vi "First_Num_from_String.vi"(1 "string":string) -> (0 "number":dbl)   [LabVIEW 2012]
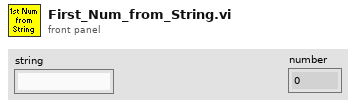
[diagram p1: front panel]
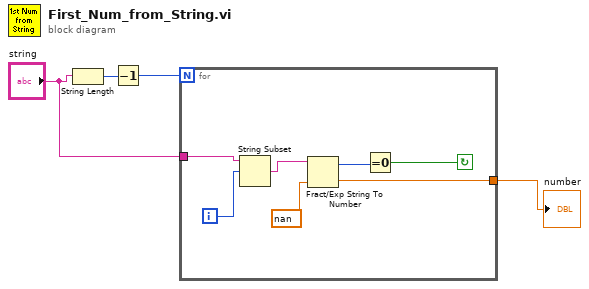
[diagram p0: block diagram]
diagram:
  n1 = String Length(string="string") -> (length=w4:i32)
  n2 = Decrement(x=w4) -> (x-1=w1:i32)
  n3 = for {
    N: w1 -> [_]
    tunnel: "string" -> [w10]
    tunnel: [w5] -> w2
    i -> [w11]
    stop <- w6 continue-if-true
    n4 = String Subset(string=w10, offset (0)=w11) -> (substring=w9:string)  [unwired: 1 in]
    n5 = Fract/Exp String To Number(string=w9, default (0 dbl)=nan ("default (0 DBL)")) -> (offset past number=w7:i32, number=w5:dbl)  [unwired: 2 in]
    n6 = Equal To 0?(x=w7) -> (x = 0?=w6:bool)
  }
  "number" <- w2
